vi "Update Displacement.vi"(11 "Element in":refnum<class "Element.lvclass">) -> (3 "Element out":refnum<class "Element.lvclass">)   [LabVIEW 2021, in "Element.lvclass"]
uses:
  Element.lvclass
  Element.lvclass/Element.ctl
  Motion/Motion.lvclass
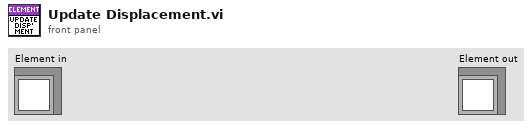
[diagram p1: front panel]
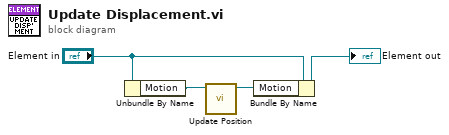
[diagram p0: block diagram]
diagram:
  n1 = Unbundle By Name("Element in") -> ("Motion"=w4:refnum<class "Motion.lvclass">)
  n2 = call "Update Position.vi"("Motion in"=w4) -> ("Motion out"=w2:refnum<class "Motion.lvclass">)  [unwired: 10 in]
  n3 = Bundle By Name(cluster="Element in", "Motion"=w2) -> (→"Element out":refnum<class "Element.lvclass">)
